vi "Lead-Lag.vi"(0 "cycle time (-1)":dbl=-1.0 format="%.2f", 2 "iteration":i32=1, 3 "Tuning Params":cluster{"Kc":dbl, "Ti":dbl, "Td":dbl}={"Kc"=1.0, "Ti"=0.01, "Td"=0.0} {"Kc" format="%.2f"; "Ti" format="%.2f"; "Td" format="%.2f"}, 4 "input (%)":dbl format="%.2f") -> (1 "output (%)":dbl format="%.2f")   [LabVIEW 2020, in "NI_PID__prctrl compat.lvlib"]
doc: "Lead/lag block, generally used as a dynamic compensator in feedforward control schemes. Input ranges between 0 and 100%; output between -100 and 200%. Lead and lag values are in minutes.\n\nThe algorithm used in this VI is a positional algorithm and is an approximation of a true exponential lead/lag.\n\nThis VI should be called from inside a while loop with a fixed cycle time. If Cycle Time is less than or equal to zero, an internal timer with 1 millisecond resolution is used for calculations. For loops that run faster than about 10 Hz, supply a cycle time in seconds.\n\nThis VI is reentrant, so you can call it from multiple, independent higher-level VIs without interference."
uses:
  NI_PID__prctrl compat.lvlib
panel:
  # "Lead-Lag Algorithm"
  # "Output  =  Gain * (S*Tlead + 1)/( S*Tlag + 1) * Input\n                Limited to +200%, -100%."
  # "Gain"
  # "Lag Time (min)"
  # "Lead Time (min)"
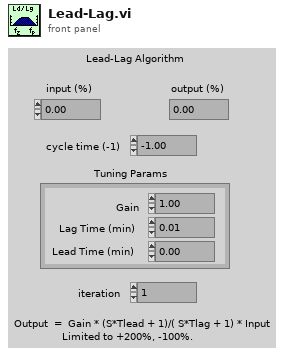
[diagram p1: front panel]
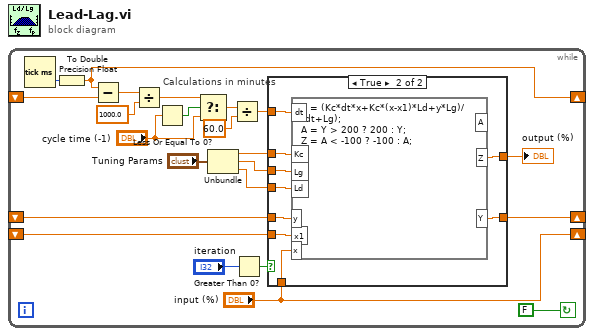
[diagram p0: block diagram]
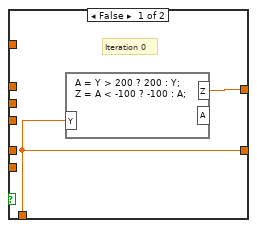
[diagram p2: hidden frame]
diagram:
  n1 = while {
    shift-left: _ -> [w14]
    shift-right: [w13] -> _
    shift-left: _ -> [w16]
    shift-right: [w17] -> _
    shift-left: _ -> [w12]
    shift-right: ["input (%)"] -> _
    stop <- FALSE continue-if-true
    n2 = Tick Count (ms)() -> (millisecond timer value=w18:u32)
    n3 = To Double Precision Float(number=w18) -> (double precision float=w17:dbl)
    n4 = Subtract(x=w17, y=w16) -> (x-y=w8:dbl)
    n5 = Divide(x=w8, y=1000.0) -> (x/y=w7:dbl)
    n6 = Less Or Equal To 0?(x="cycle time (-1)") -> (x <= 0?=w9:bool)
    n7 = Select(t=w7, s=w9, f="cycle time (-1)") -> (s? t:f=w6:dbl)
    n8 = Unbundle("Tuning Params") -> ("Kc"=w21:dbl, "Ti"=w22:dbl, "Td"=w20:dbl)
    n9 = Divide(x=w6, y=60.0) -> (x/y=w5:dbl)
    n10 = Greater Than 0?(x="iteration") -> (x > 0?=w3:bool)
    n11 = case shown="True" w3 {
      tunnel: w5 -> [_ w34]
      tunnel: w12 -> [_ w33]
      tunnel: [w24 w32] -> w13
      tunnel: w14 -> [_ w31]
      tunnel: [w25 w30] -> w15
      tunnel: w20 -> [_ w29]
      tunnel: w21 -> [_ w28]
      tunnel: w22 -> [_ w27]
      tunnel: "input (%)" -> [w24 w26]
      frame False {
        # "Iteration 0"
        n12 = formula code="A = Y > 200 ? 200 : Y;\nZ = A < -100 ? -100 : A;"("Y"=w24) -> ("Z"=w25:dbl)  [unwired: 1 out]
      }
      frame True {
        # "Calculations in minutes"
        # "Do lead/lag computation;\nLimit output to -100 to +200%"
        n13 = formula code="Y = (Kc*dt*x+Kc*(x-x1)*Ld+y*Lg)/(dt+Lg);\nA = Y > 200 ? 200 : Y;\nZ = A < -100 ? -100 : A;"("x1"=w33, "y"=w31, "x"=w26, "dt"=w34, "Ld"=w29, "Kc"=w28, "Lg"=w27) -> ("Y"=w32:dbl, "Z"=w30:dbl)  [unwired: 1 out]
      }
    }
    "output (%)" <- w15
  }
